vi "MHX Flow Properties.vi"(0 "Thermal Conductivity of FLiBe":dbl, 1 "Area":dbl, 2 "Pipe Diameter":dbl, 3 "Thermal Conductivity of FLiNaK":dbl, 4 "NDHX Tube Wall Temp":dbl, 5 "Sec Mass Flow":dbl, 6 "Average":dbl, 8 "Cp of FLiNaK":dbl, 9 "MHX Tube Wall Temp":dbl, 10 "FLiNaK Ave Viscosity":dbl, 11 "Pri Mass Flow":dbl, 12 "Specific Heat Capacity of FLiBe":dbl) -> (16 "MHX Pri Re":dbl, 18 "FLiBe Average Viscosity (Pa-s)":dbl, 20 "FLiBe Wall Viscosity (Pa-s)":dbl, 21 "MHX Sec Re":dbl, 22 "MHX Pri Phi":dbl, 23 "MHX Pri Pr":dbl, 24 "MHX Sec Phi":dbl, 25 "MHX Sec Pr":dbl, 26 "Sec Mass Flux (kg/s-m^2)":dbl)   [LabVIEW 2019]
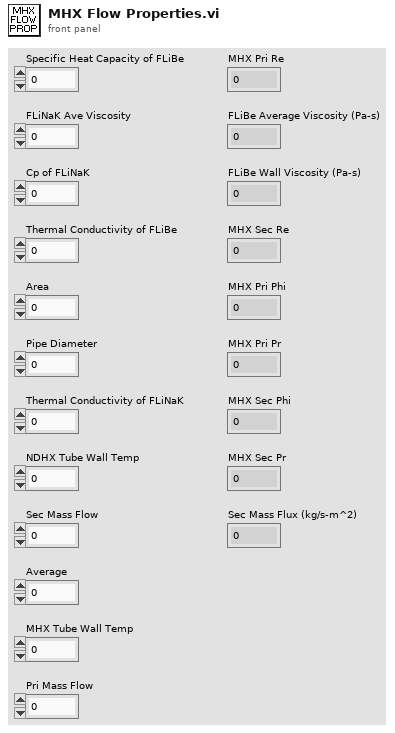
[diagram p1: front panel]
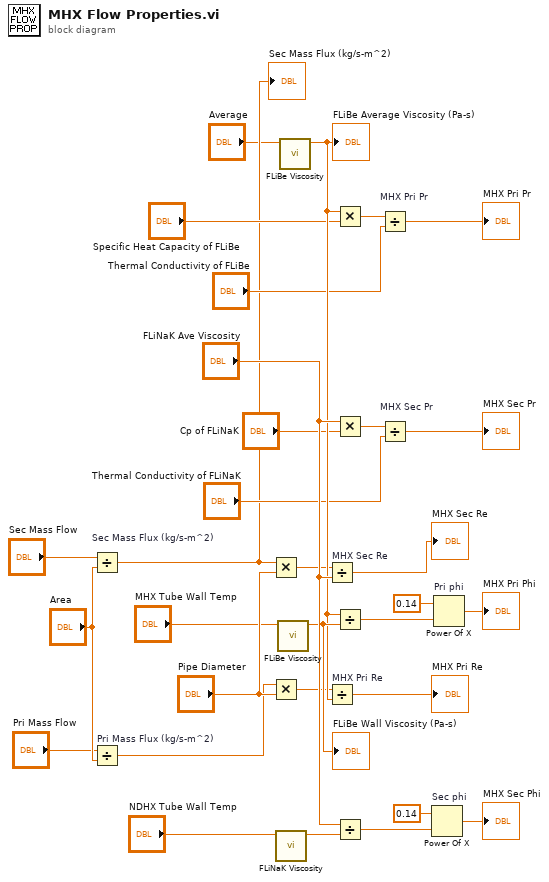
[diagram p0: block diagram]
diagram:
  n1 = Divide "Sec Mass Flux (kg/s-m^2)"(x="Sec Mass Flow", y="Area") -> (x/y=w9:dbl)
  "Sec Mass Flux (kg/s-m^2)" <- w9
  n2 = Divide "Pri Mass Flux (kg/s-m^2)"(x="Pri Mass Flow", y="Area") -> (x/y=w8:dbl)
  n3 = Multiply(x=w9, y="Pipe Diameter") -> (x*y=w7:dbl)
  n4 = Multiply(x=w8, y="Pipe Diameter") -> (x*y=w6:dbl)
  n5 = call "FLiNaK Viscosity.vi"("Temperature (K)"="NDHX Tube Wall Temp") -> ("FLiNaK Viscosity (Pa-s)"=w25:dbl)  [unwired: 10 in]
  n6 = call "FLiBe Viscosity.vi"("Temperature (K)"="MHX Tube Wall Temp") -> ("FLiBe Viscosity (Pa-s)"=w18:dbl)  [unwired: 10 in]
  "FLiBe Wall Viscosity (Pa-s)" <- w18
  n7 = call "FLiBe Viscosity.vi"("Temperature (K)"="Average") -> ("FLiBe Viscosity (Pa-s)"=w17:dbl)  [unwired: 10 in]
  "FLiBe Average Viscosity (Pa-s)" <- w17
  n8 = Divide "MHX Sec Re"(x=w7, y="FLiNaK Ave Viscosity") -> (x/y=→"MHX Sec Re":dbl)
  n9 = Divide "MHX Pri Re"(x=w6, y=w17) -> (x/y=→"MHX Pri Re":dbl)
  n10 = Multiply(x=w17, y="Specific Heat Capacity of FLiBe") -> (x*y=w11:dbl)
  n11 = Multiply(x="FLiNaK Ave Viscosity", y="Cp of FLiNaK") -> (x*y=w12:dbl)
  n12 = Divide(x=w17, y=w18) -> (x/y=w19:dbl)
  n13 = Divide(x="FLiNaK Ave Viscosity", y=w25) -> (x/y=w22:dbl)
  n14 = Divide "MHX Pri Pr"(x=w11, y="Thermal Conductivity of FLiBe") -> (x/y=→"MHX Pri Pr":dbl)
  n15 = Divide "MHX Sec Pr"(x=w12, y="Thermal Conductivity of FLiNaK") -> (x/y=→"MHX Sec Pr":dbl)
  n16 = Power Of X "Sec phi"(1:w22, 2:0.14 ("y")) -> (0:→"MHX Sec Phi":dbl)
  n17 = Power Of X "Pri phi"(1:w19, 2:0.14 ("y")) -> (0:→"MHX Pri Phi":dbl)
